vi "DefBallTrajSkill.vi"(8 "error in (no error)":errorcluster, 9 "Robot":refnum<class "Robot.lvclass">, 10 "Game":refnum<class "Game.lvclass">, 11 "DefBallTrajSkill in":refnum<class "DefBallTrajSkill.lvclass">) -> (0 "error out":errorcluster, 2 "robot out":refnum<class "Robot.lvclass">, 3 "DefBallTrajSkill out":refnum<class "DefBallTrajSkill.lvclass">)   [LabVIEW 2018, in "DefBallTrajSkill.lvclass"]
uses:
  DefBallTrajSkill.lvclass
  Game_class/Game.lvclass
  Robot_class/Robot.lvclass
  Game_class/Game.lvclass/Game.ctl
  Object_class/Object.lvclass/Object.ctl
  Ball_class/Ball.lvclass/Ball.ctl
  Robot_class/Robot.lvclass/Robot.ctl
  Game_class/Read BallRef.vi
  Game_class/Read FieldRef.vi
  Object_class/Read x.vi
  Object_class/Read y.vi
  Ball_class/Read v_x.vi
  Ball_class/Read v_y.vi
  Robot_class/Write dest_x.vi
  Robot_class/Write dest_y.vi
  Robot_class/Write dest_orientation.vi
  Ball_class/Ball.lvclass
  C:/Users/lucas/Documents/RoboIME/SSL_AI - newGoalie/Object_class/Object.lvclass
  Field_class/Field.lvclass
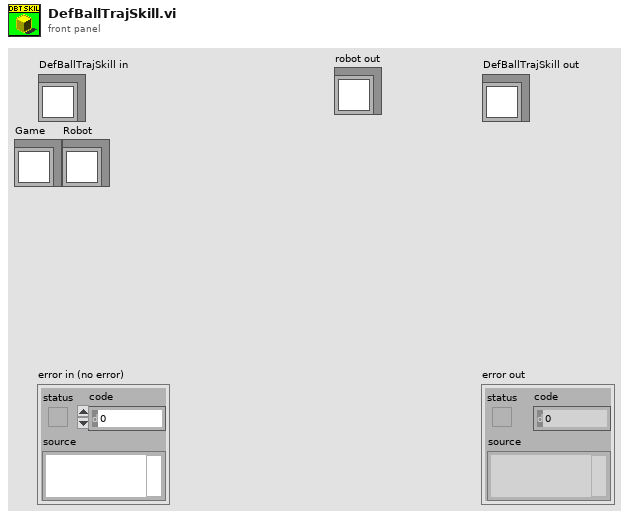
[diagram p1: front panel]
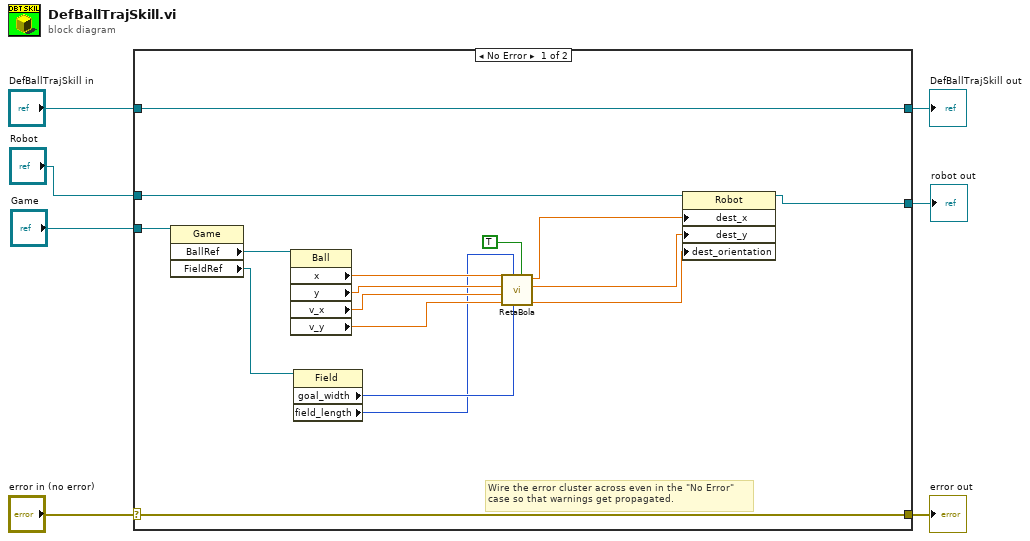
[diagram p0: block diagram]
diagram:
  n1 = case shown="No Error" "error in (no error)" {
    selector: "error in (no error)" -> [w23 w26]
    tunnel: [w23 w26] -> w6
    tunnel: [w24 w25] -> w4
    tunnel: "DefBallTrajSkill in" -> [w24 w25]
    tunnel: "Game" -> [w22 _]
    tunnel: "Robot" -> [w12 _]
    tunnel: [w8 _] -> w1
    frame No Error {
      # "Wire the error cluster across even in the \"No Error\"\ncase so that warnings get propagated."
      n2 = property class="Game"(reference=w22) -> ("BallRef"=w21:refnum<class "Ball.lvclass">, "FieldRef"=w16:refnum<class "Field.lvclass">)  [unwired: 1 in, 2 out]
      n3 = property class="Ball"(reference=w21) -> ("x"=w20:dbl, "y"=w19:dbl, "v_x"=w18:dbl, "v_y"=w17:dbl)  [unwired: 1 in, 2 out]
      n4 = property class="Field"(reference=w16) -> ("goal_width"=w15:i32, "field_length"=w14:i32)  [unwired: 1 in, 2 out]
      n5 = call "RetaBola.vi"("Meio?"=TRUE, "Goal Width"=w15, "Field Lenght"=w14, "Vy bola"=w17, "Vx bola"=w18, "Y bola"=w19, "X bola"=w20) -> ("Orientação"=w9:dbl, "Y goleiro"=w10:dbl, "X goleiro"=w11:dbl)  [unwired: 2 in]
      n6 = property class="Robot"(reference=w12, "dest_x"=w11, "dest_y"=w10, "dest_orientation"=w9) -> (reference out=w8:refnum<class "Robot.lvclass">)  [unwired: 1 in, 1 out]
    }
    frame Error {
    }
  }
  "error out" <- w6
  "DefBallTrajSkill out" <- w4
  "robot out" <- w1
